vi "getMonos.vi"(8 "error in (no error)":errorcluster, 11 "Monochromator in":refnum<class "Monochromator.lvclass">) -> (0 "error out":errorcluster, 1 "Current UniqueID":string="Mono4", 2 "Mono ID":string(combo)="Mono4", 3 "Monochromator out":refnum<class "Monochromator.lvclass">, 4 "Monos":cluster{"String":string, "String":string}[](array[cluster]))   [LabVIEW 2016, in "Monochromator.lvclass"]
uses:
  Monochromator.lvclass
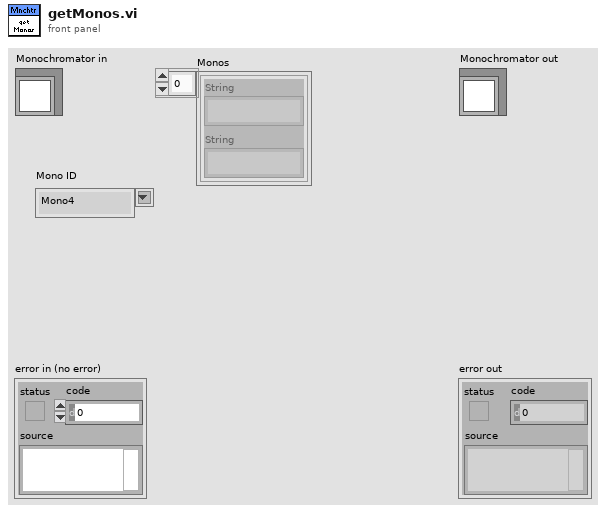
[diagram p1: front panel]
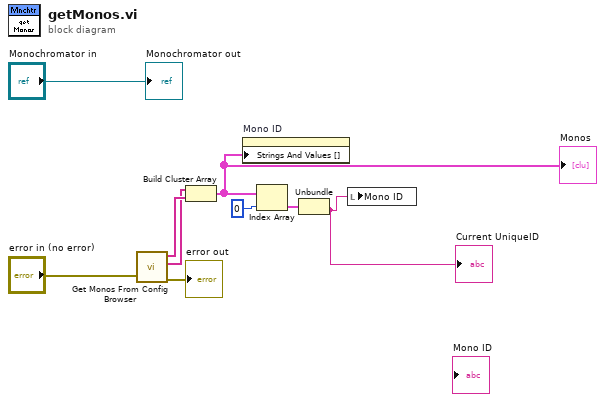
[diagram p0: block diagram]
diagram:
  n1 = call "Get Monos From Config Browser.vi"("error in (no error)"="error in (no error)") -> ("UniqueIDs"=w5:string[], "Mono ID"=w4:string[], "error out"=→"error out":errorcluster)  [unwired: 2 in]
  n2 = Build Cluster Array(w4, w5) -> (w7:cluster{"String":string, "String":string}[])
  "Monos" <- w7
  n3 = property on="Mono ID" class="CmbBox"("Strings And Values []"=w7) -> ()  [unwired: 2 in, 2 out]
  n4 = Index Array(array=w7, index=0) -> (element=w6:cluster{"String":string, "String":string})
  n5 = Unbundle(w6) -> ("String"=w1:string)  [unwired: 1 out]
  "Current UniqueID" <- w1
  n6 = local write "Mono ID"(w1) -> ()
  "Monochromator out" <- "Monochromator in"
